vi "Sound_gen3.vi"(5 "Sound/Pause":bool, 6 "Sound time(s)":dbl=1.0, 7 "Dit time(ms)":u32, 8 "stop":bool, 9 "Sound On/Off":bool=TRUE, 10 "Frequency":dbl, 11 "Volume":dbl(knob) scale=0.0..100.0) -> ()   [LabVIEW 2022 SP3]
uses:
  <vilib>/sound2/lvsound2.llb/Sound Data Format.ctl
  <vilib>/sound2/lvsound2.llb/Sampling Mode.ctl
  <vilib>/sound2/lvsound2.llb/Sound Output Write (DBL Single).vi
  <vilib>/sound2/lvsound2.llb/Sound Output Set Volume (Single).vi
panel:
  out "error out":errorcluster
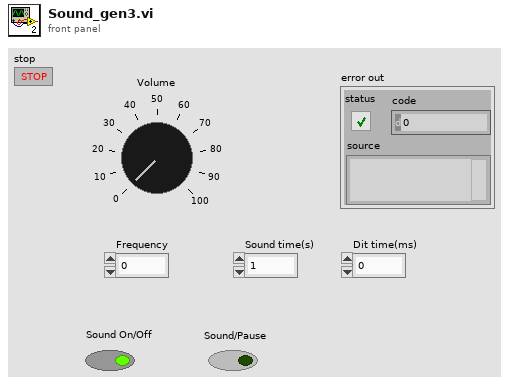
[diagram p1: front panel]
types:
  T1 = typedef "Sound Data Format.ctl" = cluster{"sample rate (S/s)":dbl, "number of channels":i32, "bits per sample":i32}
  T2 = typedef "Sampling Mode.ctl" = i32
  T3 = typedef "Sound Output Task ID.ctl" = u32
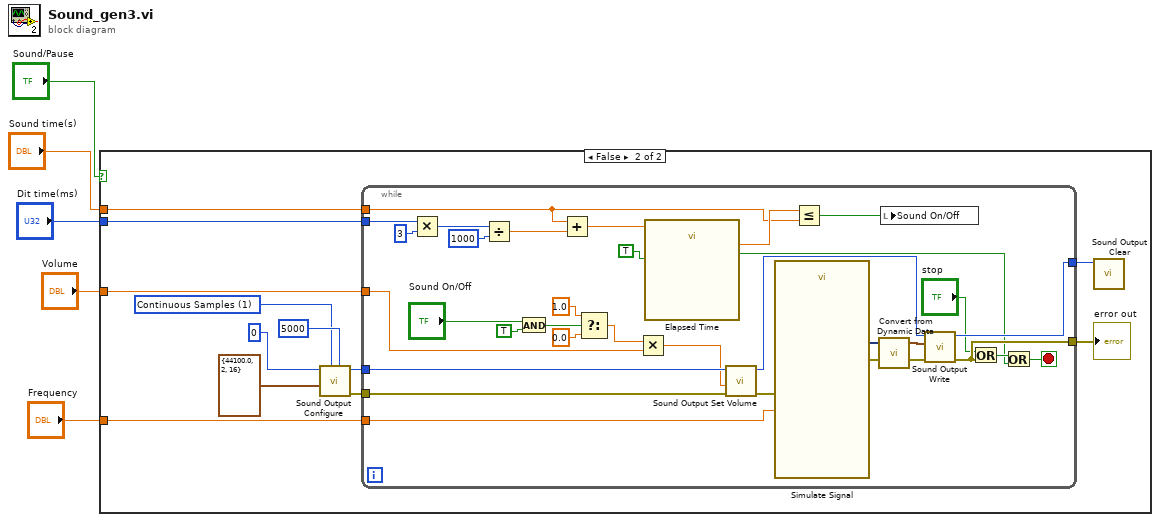
[diagram p0: block diagram]
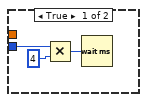
[diagram p2: hidden frame]
diagram:
  n1 = case shown="False" "Sound/Pause" {
    tunnel: "Sound time(s)" -> [_ w12]
    tunnel: "Dit time(ms)" -> [w8 w11]
    tunnel: "Frequency" -> [_ w10]
    tunnel: "Volume" -> [_ w9]
    frame True {
      n2 = Multiply(x=w8, y=u32 4) -> (x*y=w6:u32)
      n3 = Wait (ms)(milliseconds to wait=w6) -> ()  [unwired: 1 out]
    }
    frame False {
      w15 = T2 1 items=["Finite Samples", "Continuous Samples"] ("sample mode")
      n4 = call <vilib>:"Sound Output Configure.vi"("number of samples/ch"=5000, "sample mode"=w15, "sound format"=T1 {"sample rate (S/s)"=44100.0, "number of channels"=2, "bits per sample"=16}, "device ID"=u32 0) -> ("error out"=w18:errorcluster, "task ID"=w17:T3)  [unwired: 6 in]
      n5 = while {
        tunnel: w17 -> [w52]
        tunnel: [w49] -> w20
        tunnel: w18 -> [w51]
        tunnel: [w50] -> w19
        tunnel: w12 -> [w23]
        tunnel: w11 -> [w32]
        tunnel: w10 -> [w22]
        tunnel: w9 -> [w21]
        stop <- w33 stop-if-true
        n6 = Multiply(x=w32, y=u32 3) -> (x*y=w26:u32)
        n7 = Divide(x=w26, y=u32 1000 ("x")) -> (x/y=w24:dbl)
        n8 = And(x="Sound On/Off", y=TRUE) -> (x .and. y?=w41:bool)
        n9 = Add(x=w23, y=w24) -> (x+y=w29:dbl)
        n10 = Select(t=1.0, s=w41, f=0.0) -> (s? t:f=w38:dbl)
        n11 = Multiply(x=w38, y=w21) -> (x*y=w37:dbl)
        n12 = call "Elapsed Time"("Time Target (s)"=w29, "Auto Reset"=TRUE) -> ("Elapsed Time (s)"=w28:dbl, "Time has Elapsed"=w30:bool)  [unwired: 10 in, 6 out]
        n13 = call-poly <vilib>:"Sound Output Set Volume.vi"("error in (no error)"=w51, "volume"=w37, "task ID"=w52) -> ("error out"=w48:errorcluster, "task ID out"=w46:T3)  [unwired: 7 in]
        n14 = call "Simulate Signal"("Frequency"=w22, "error in (no error)"=w48) -> ("Sine"=w47:dynamicdata, "error out"=w44:errorcluster)  [unwired: 12 in]
        n15 = Less Or Equal?(x=w28, y=w23) -> (x <= y?=w27:bool)
        n16 = call "Convert from Dynamic Data"("Dynamic Data Type"=w47) -> ("Waveform"=w45:waveform(dbl))  [unwired: 3 in]
        n17 = local write "Sound On/Off"(w27) -> ()
        n18 = call-poly <vilib>:"Sound Output Write.vi"("error in (no error)"=w44, "data"=w45, "task ID"=w46) -> ("error out"=w50:errorcluster, "task ID out"=w49:T3)  [unwired: 7 in]
        n19 = Or(x="stop", y=w50) -> (x .or. y?=w34:bool)
        n20 = Or(x=w34, y=w30) -> (x .or. y?=w33:bool)
      }
      "error out" <- w19
      n21 = call <vilib>:"Sound Output Clear.vi"("task ID"=w20) -> ()  [unwired: 10 in, 1 out]
    }
  }
